vi "MaterialCharacterization.vi"(8 "error in":errorcluster) -> (0 "error out":errorcluster)   [LabVIEW 2013, in "MaterialCharacterization.lvlib"]
uses:
  MaterialCharacterization.lvlib
  Sources/Main/Options.ctl
  Sources/Main/Measurement-types.ctl
  Sources/Main/Main-actions.ctl
  Sources/Main/MC-Main.lvclass/MC-Main.ctl
  Sources/Main/Enqueue-modes.ctl
  Sources/UI/Pane-names.ctl
  Sources/Main/Write Measurement type.vi
  Sources/Main/Write Scan file path.vi
  Sources/Main/Read UI.vi
  Sources/UI/MC-UI.lvclass
  Sources/Main/MC-Main.lvclass
panel:
  in  "Measurement settings":bool
  in  "Select measurement":T1
  in  "Load configuration":bool
  in  "Stop":bool
  in  "Save configuration":bool
  in  "Activate":bool
  in  "Start":bool
  in  "Help":bool
  in  "View raw path":bool
  in  "SM1000 scan file":path
  in  "View scan file":bool
  in  "Options":T2
  out "Data table":string[][](table)
  out "Status":string caption="Status:"
  out "Action":string caption="Action:"
  # "Config"
  # "Exec"
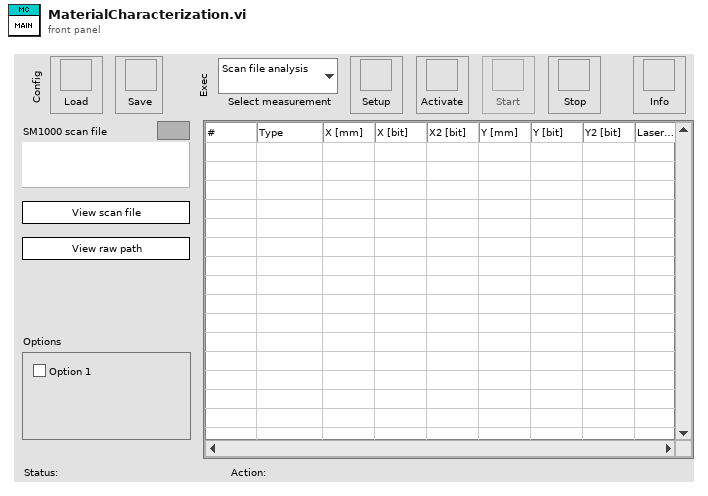
[diagram p1: front panel]
types:
  T1 = typedef "MaterialCharacterization.lvlib/MC-Main.lvclass/Measurement-types.ctl" = enum16{"Scan file analysis", "Thermal conductivity", "Laser reflection", "Combined"}
  T2 = typedef "MaterialCharacterization.lvlib/MC-Main.lvclass/Options.ctl" = cluster{"Option 1":bool}
  T3 = typedef "MaterialCharacterization.lvlib/MC-Main.lvclass/Main-actions.ctl" = enum16{"Idle", "Initialize", "Load configuration", "Save configuration", "Load file", "Edit settings", "View scan file", "View raw path", "Edit measurement settings", "Activate", "Start", "Stop", "Refresh display", "Exit"}
  T4 = typedef "MaterialCharacterization.lvlib/MC-Main.lvclass/Object-reference.ctl" = refnum<data-value>
  T5 = typedef "MaterialCharacterization.lvlib/MC-Main.lvclass/Enqueue-modes.ctl" = enum16{"Default", "Priority", "Flush"}
  T6 = typedef "MaterialCharacterization.lvlib/MC-UI.lvclass/Pane-names.ctl" = enum16{"Toolbar", "Help bar", "Toolbar lower border", "Center panel", "Main panel", "Settings panel", "Status bar upper border", "General state bar", "Information bar"}
  T7 = typedef "MaterialCharacterization.lvlib/MC-UI.lvclass/Panes-reference.ctl" = refnum<data-value>
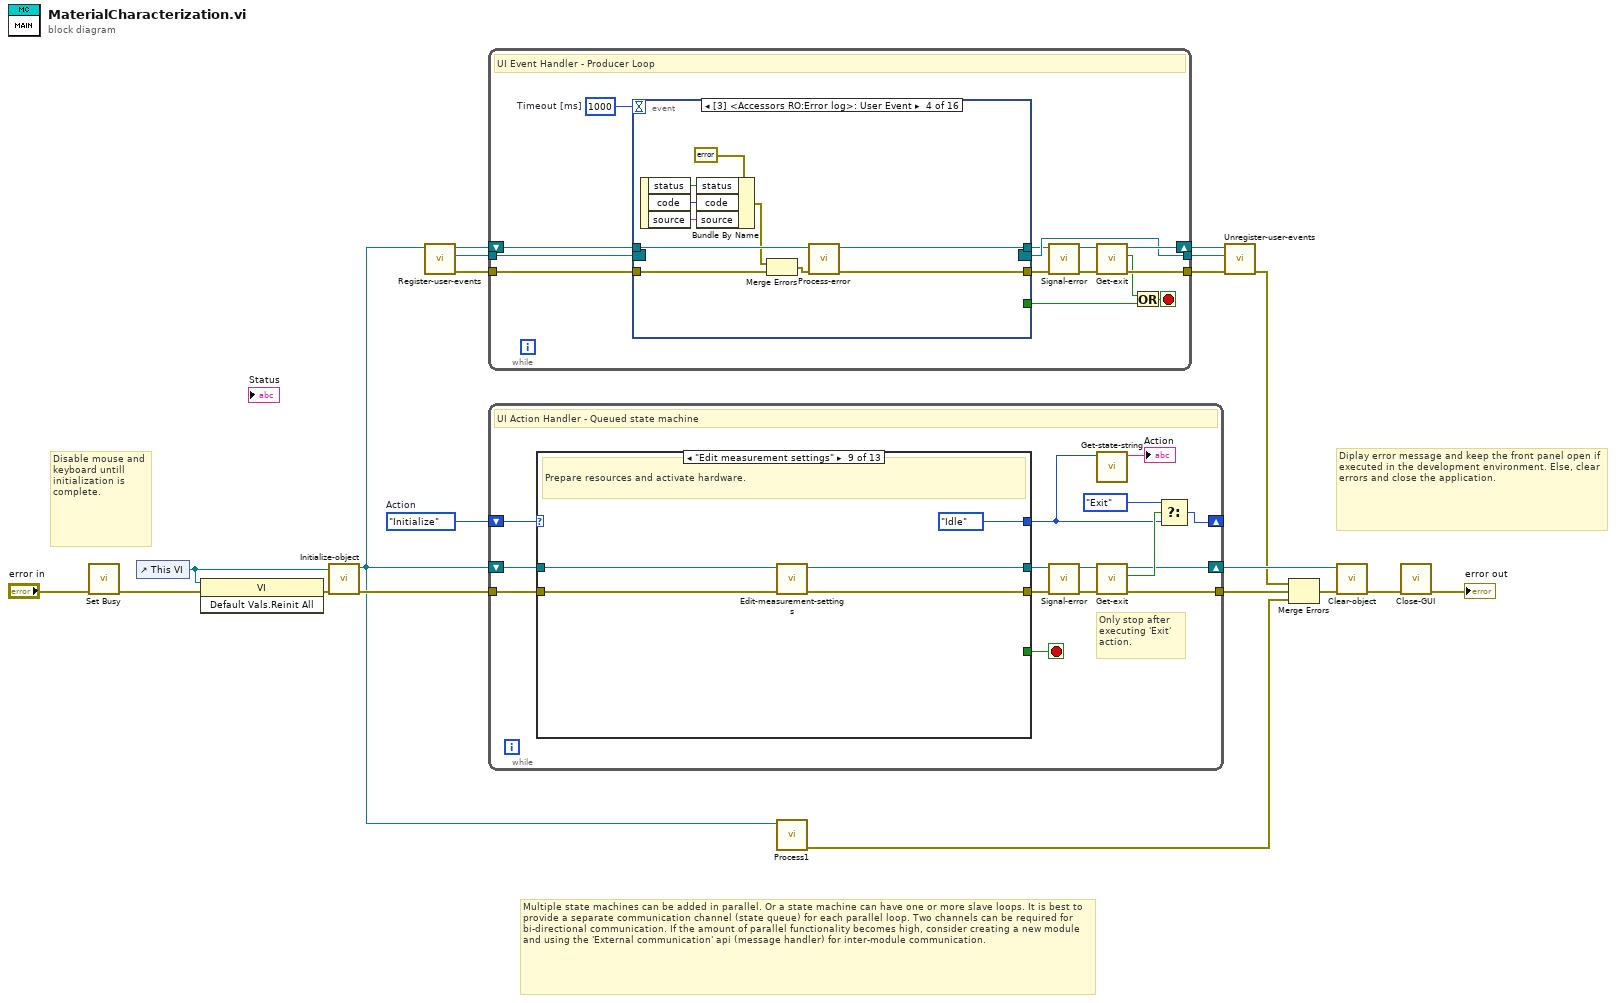
[diagram p0: block diagram]
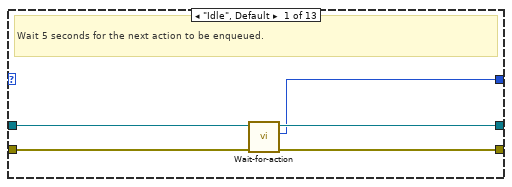
[diagram p2: hidden frame]
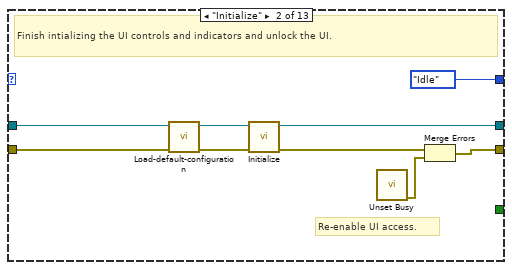
[diagram p3: hidden frame]
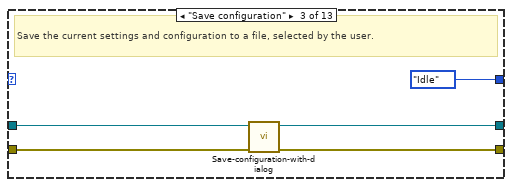
[diagram p4: hidden frame]
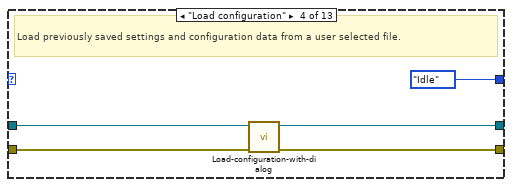
[diagram p5: hidden frame]
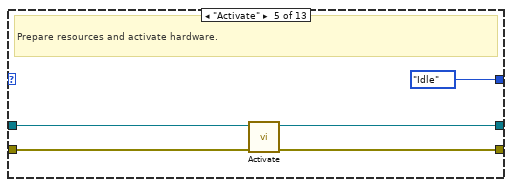
[diagram p6: hidden frame]
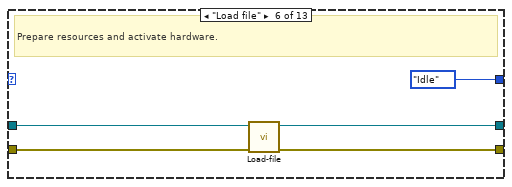
[diagram p7: hidden frame]
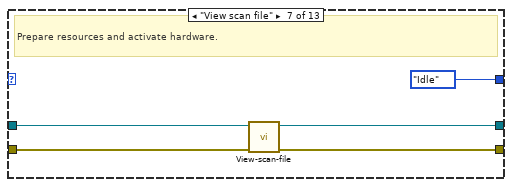
[diagram p8: hidden frame]
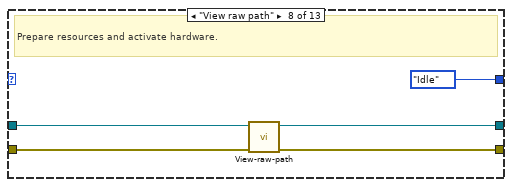
[diagram p9: hidden frame]
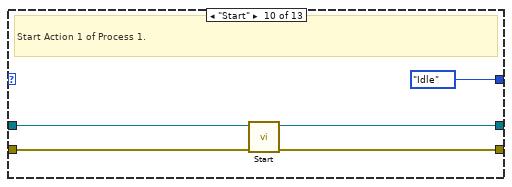
[diagram p10: hidden frame]
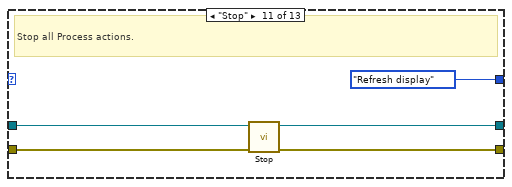
[diagram p11: hidden frame]
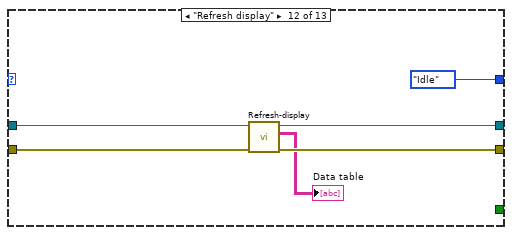
[diagram p12: hidden frame]
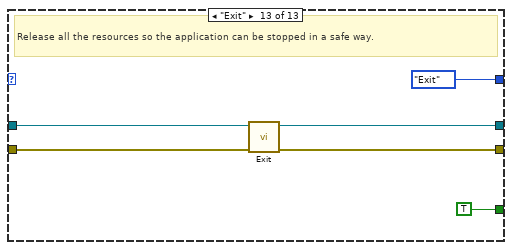
[diagram p13: hidden frame]
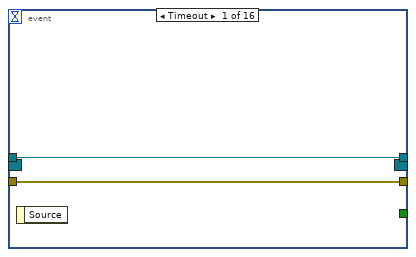
[diagram p14: hidden frame]
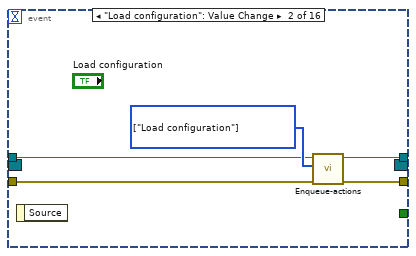
[diagram p15: hidden frame]
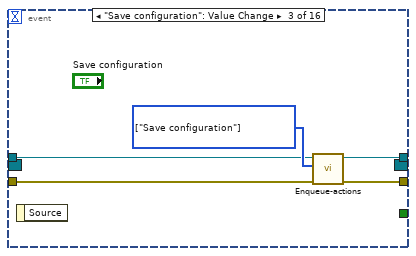
[diagram p16: hidden frame]
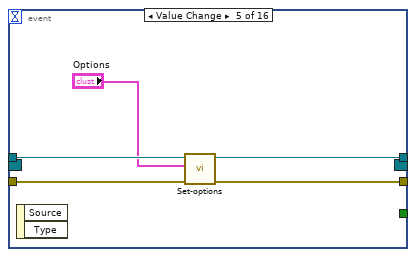
[diagram p17: hidden frame]
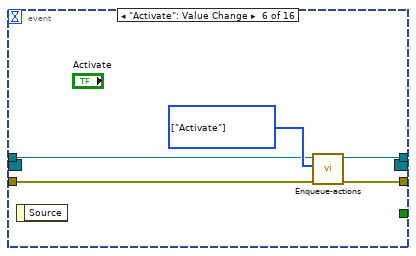
[diagram p18: hidden frame]
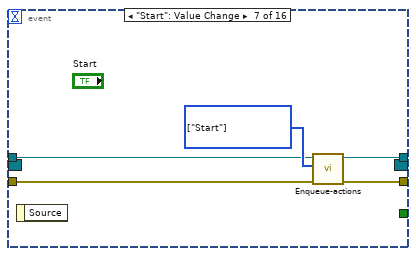
[diagram p19: hidden frame]
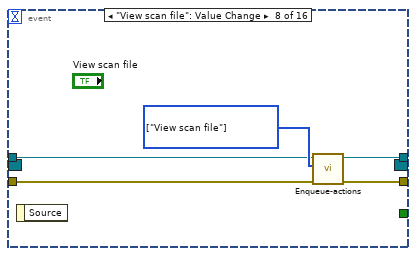
[diagram p20: hidden frame]
diagram:
  w20 = Main-actions."Initialize"  # Action
  # "Multiple state machines can be added in parallel. Or a state machine can have one or more slave loops. It is best to provide a separate communication channel (state queue) for each parallel loop. Two channels can be required for bi-directional communication. If the amount of parallel functionality becomes high, consider creating a new module and using the 'External communication' api (message handler) for inter-module communication."
  # "Disable mouse and keyboard untill initialization is complete."
  # "Diplay error message and keep the front panel open if executed in the development environment. Else, clear errors and close the application."
  n1 = call <vilib>:"Set Busy.vi"("error in (no error)"="error in") -> ("error out"=w3:errorcluster)  [unwired: 9 in, 1 out]
  n2 = control-ref of="This VI"() -> (w2:refnum<vi>)
  n3 = invoke class="VI" method="Default Vals.Reinit All"(reference=w2, error in=w3) -> (error out=w1:errorcluster)  [unwired: 1 in, 2 out]
  n4 = call "Initialize-object.vi"("Main VI ref"=w2, "error in (no error)"=w1) -> ("error out"=w13:errorcluster, "Object ref out"=w4:T4)  [unwired: 8 in]
  n5 = call "Register-user-events.vi"("Object ref in"=w4) -> ("error out"=w10:errorcluster, "Event registration"=w9:refnum<event-registration>, "Object ref out"=w11:T4)  [unwired: 8 in]
  n6 = while {
    shift-right: [w29] -> w6
    shift-left: w11 -> [w32]
    tunnel: w9 -> [w27]
    tunnel: [w26] -> w5
    tunnel: w10 -> [w33]
    tunnel: [w28] -> w8
    stop <- w23 stop-if-true
    w34 = 1000  # Timeout [ms]
    # "UI Event Handler - Producer Loop"
    n7 = event shown="[3] <Accessors RO:Error log>: User Event" {
      selector: w27 -> [_ _ _ _ _ _ _ _ _ _ _ _ _ _ _ _]
      dyn-events: [_ _ _ _ _ _ _ _ _ _ _ _ _ _ _ _] -> w26
      timeout: w34 -> [_ _ _ _ _ _ _ _ _ _ _ _ _ _ _ _]
      tunnel: w33 -> [w36 w41 w46 w54 w59 w66 w71 w76 w81 w86 w89 w92 w105 w108 w112 w156]
      tunnel: [w36 w40 w45 w53 w60 w65 w70 w75 w80 w85 w88 w95 w104 w108 w110 w161] -> w24
      tunnel: w32 -> [w35 w38 w43 w56 w58 w63 w68 w73 w78 w83 w91 w93 w102 w106 w113 w157]
      tunnel: [w35 w37 w42 w55 w61 w62 w67 w72 w77 w82 w90 w97 w101 w106 w111 w158] -> w25
      tunnel: [_ _ _ _ _ _ _ _ _ _ _ _ _ _ _ TRUE] -> w21
      event Timeout {
        n8 = event-data() -> ()  [unwired: 1 in, 1 out]
      }
      event "Load configuration": Value Change {
        w39 = T3[] [enum."Load configuration"] items=["Idle", "Initialize", "Load configuration", "Save configuration", "Load file", "Edit settings", "View scan file", "View raw path", "Edit measurement settings", "Activate", "Start", "Stop", "Refresh display", "Exit"] ("State array")
        n9 = event-data() -> ()  [unwired: 1 in, 1 out]
        n10 = call "Enqueue-actions.vi"("error in (no error)"=w41, "State array"=w39, "State queue in"=w38) -> ("error out"=w40:errorcluster, "State queue out"=w37:T4)  [unwired: 6 in, 1 out]
      }
      event "Save configuration": Value Change {
        w44 = T3[] [enum."Save configuration"] items=["Idle", "Initialize", "Load configuration", "Save configuration", "Load file", "Edit settings", "View scan file", "View raw path", "Edit measurement settings", "Activate", "Start", "Stop", "Refresh display", "Exit"] ("State array")
        n11 = event-data() -> ()  [unwired: 1 in, 1 out]
        n12 = call "Enqueue-actions.vi"("error in (no error)"=w46, "State array"=w44, "State queue in"=w43) -> ("error out"=w45:errorcluster, "State queue out"=w42:T4)  [unwired: 6 in, 1 out]
      }
      event User Event {
        n13 = event-data() -> ("status"=w51:bool, "code"=w50:i32, "source"=w49:string)  [unwired: 1 in]
        n14 = Bundle By Name(cluster=errorcluster {"status"=FALSE, "code"=0, "source"=""} ("error constant"), "status"=w51, "code"=w50, "source"=w49) -> (w47:errorcluster)
        n15 = Merge Errors(w47, w54) -> (w48:errorcluster)
        n16 = call "Process-error.vi"("error in (no error)"=w48, "Data in"=w56) -> ("error out"=w53:errorcluster, "Data out"=w55:T4)  [unwired: 8 in]
      }
      event Value Change {
        n17 = event-data() -> ()  [unwired: 1 in, 2 out]
        n18 = call "Set-options.vi"("error in (no error)"=w59, "Options"="Options", "Object ref in"=w58) -> ("error out"=w60:errorcluster, "Object ref out"=w61:T4)  [unwired: 7 in]
      }
      event "Activate": Value Change {
        w64 = T3[] [enum."Activate"] items=["Idle", "Initialize", "Load configuration", "Save configuration", "Load file", "Edit settings", "View scan file", "View raw path", "Edit measurement settings", "Activate", "Start", "Stop", "Refresh display", "Exit"] ("State array")
        n19 = event-data() -> ()  [unwired: 1 in, 1 out]
        n20 = call "Enqueue-actions.vi"("error in (no error)"=w66, "State array"=w64, "State queue in"=w63) -> ("error out"=w65:errorcluster, "State queue out"=w62:T4)  [unwired: 6 in, 1 out]
      }
      event "Start": Value Change {
        w69 = T3[] [enum."Start"] items=["Idle", "Initialize", "Load configuration", "Save configuration", "Load file", "Edit settings", "View scan file", "View raw path", "Edit measurement settings", "Activate", "Start", "Stop", "Refresh display", "Exit"] ("State array")
        n21 = event-data() -> ()  [unwired: 1 in, 1 out]
        n22 = call "Enqueue-actions.vi"("error in (no error)"=w71, "State array"=w69, "State queue in"=w68) -> ("error out"=w70:errorcluster, "State queue out"=w67:T4)  [unwired: 6 in, 1 out]
      }
      event "View scan file": Value Change {
        w74 = T3[] [enum."View scan file"] items=["Idle", "Initialize", "Load configuration", "Save configuration", "Load file", "Edit settings", "View scan file", "View raw path", "Edit measurement settings", "Activate", "Start", "Stop", "Refresh display", "Exit"] ("State array")
        n23 = event-data() -> ()  [unwired: 1 in, 1 out]
        n24 = call "Enqueue-actions.vi"("error in (no error)"=w76, "State array"=w74, "State queue in"=w73) -> ("error out"=w75:errorcluster, "State queue out"=w72:T4)  [unwired: 6 in, 1 out]
      }
      event "View raw path": Value Change {
        w79 = T3[] [enum."View raw path"] items=["Idle", "Initialize", "Load configuration", "Save configuration", "Load file", "Edit settings", "View scan file", "View raw path", "Edit measurement settings", "Activate", "Start", "Stop", "Refresh display", "Exit"] ("State array")
        n25 = event-data() -> ()  [unwired: 1 in, 1 out]
        n26 = call "Enqueue-actions.vi"("error in (no error)"=w81, "State array"=w79, "State queue in"=w78) -> ("error out"=w80:errorcluster, "State queue out"=w77:T4)  [unwired: 6 in, 1 out]
      }
      event "Measurement settings": Value Change {
        w84 = T3[] [enum."Edit measurement settings"] items=["Idle", "Initialize", "Load configuration", "Save configuration", "Load file", "Edit settings", "View scan file", "View raw path", "Edit measurement settings", "Activate", "Start", "Stop", "Refresh display", "Exit"] ("State array")
        n27 = event-data() -> ()  [unwired: 1 in, 1 out]
        n28 = call "Enqueue-actions.vi"("error in (no error)"=w86, "State array"=w84, "State queue in"=w83) -> ("error out"=w85:errorcluster, "State queue out"=w82:T4)  [unwired: 6 in, 1 out]
      }
      event Value Change {
        n29 = event-data() -> ()  [unwired: 1 in, 2 out]
        n30 = property class="MC-Main.lvclass"(reference=w91, error in=w89, "Accessors/Modifiers:V Measurement type"="Select measurement") -> (reference out=w90:T4, error out=w88:errorcluster)
      }
      event "SM1000 scan file": Value Change {
        w94 = T3[] [enum."Load file"] items=["Idle", "Initialize", "Load configuration", "Save configuration", "Load file", "Edit settings", "View scan file", "View raw path", "Edit measurement settings", "Activate", "Start", "Stop", "Refresh display", "Exit"] ("State array")
        n31 = event-data() -> ()  [unwired: 1 in, 2 out]
        n32 = property class="MC-Main.lvclass"(reference=w93, error in=w92, "Accessors/Modifiers:V Scan file path"="SM1000 scan file") -> (reference out=w98:T4, error out=w96:errorcluster)
        n33 = call "Enqueue-actions.vi"("error in (no error)"=w96, "State array"=w94, "State queue in"=w98) -> ("error out"=w95:errorcluster, "State queue out"=w97:T4)  [unwired: 6 in, 1 out]
      }
      event "Stop": Value Change {
        w103 = T3[] [enum."Stop"] items=["Idle", "Initialize", "Load configuration", "Save configuration", "Load file", "Edit settings", "View scan file", "View raw path", "Edit measurement settings", "Activate", "Start", "Stop", "Refresh display", "Exit"] ("State array")
        n34 = event-data() -> ()  [unwired: 1 in, 1 out]
        n35 = call "Enqueue-actions.vi"("Enqueue mode"=Enqueue-modes."Flush", "error in (no error)"=w105, "State array"=w103, "State queue in"=w102) -> ("error out"=w104:errorcluster, "State queue out"=w101:T4)  [unwired: 5 in, 1 out]
      }
      event "Help": Value Change {
        # "Toggle the visibility of the context help window."
        n36 = event-data() -> ()  [unwired: 1 in, 1 out]
        n37 = Control Help Window(1:"Help") -> ()  [unwired: 1 in]
      }
      event Menu Selection (User) {
        n38 = event-data() -> ("ItemTag"=w109:string)  [unwired: 1 in, 1 out]
        n39 = case shown="\"TOOLBAR\"" w109 {
          tunnel: w113 -> [w115 w119 w124 w129 w134 w139 w147 w154]
          tunnel: w112 -> [w114 w117 w122 w127 w132 w137 w143 w150]
          tunnel: [w115 w118 w123 w128 w133 w138 w146 w153] -> w111
          tunnel: [w114 w116 w121 w126 w131 w136 w145 w152] -> w110
          frame Default {
          }
          frame "LOAD_CONFIG" {
            w120 = T3[] [enum."Load configuration"] items=["Idle", "Initialize", "Load configuration", "Save configuration", "Load file", "Edit settings", "View scan file", "View raw path", "Edit measurement settings", "Activate", "Start", "Stop", "Refresh display", "Exit"] ("State array")
            n40 = call "Enqueue-actions.vi"("error in (no error)"=w117, "State array"=w120, "State queue in"=w119) -> ("error out"=w116:errorcluster, "State queue out"=w118:T4)  [unwired: 6 in, 1 out]
          }
          frame "SAVE_CONFIG" {
            w125 = T3[] [enum."Save configuration"] items=["Idle", "Initialize", "Load configuration", "Save configuration", "Load file", "Edit settings", "View scan file", "View raw path", "Edit measurement settings", "Activate", "Start", "Stop", "Refresh display", "Exit"] ("State array")
            n41 = call "Enqueue-actions.vi"("error in (no error)"=w122, "State array"=w125, "State queue in"=w124) -> ("error out"=w121:errorcluster, "State queue out"=w123:T4)  [unwired: 6 in, 1 out]
          }
          frame "ACTIVATE" {
            w130 = T3[] [enum."Activate"] items=["Idle", "Initialize", "Load configuration", "Save configuration", "Load file", "Edit settings", "View scan file", "View raw path", "Edit measurement settings", "Activate", "Start", "Stop", "Refresh display", "Exit"] ("State array")
            n42 = call "Enqueue-actions.vi"("error in (no error)"=w127, "State array"=w130, "State queue in"=w129) -> ("error out"=w126:errorcluster, "State queue out"=w128:T4)  [unwired: 6 in, 1 out]
          }
          frame "START" {
            w135 = T3[] [enum."Start"] items=["Idle", "Initialize", "Load configuration", "Save configuration", "Load file", "Edit settings", "View scan file", "View raw path", "Edit measurement settings", "Activate", "Start", "Stop", "Refresh display", "Exit"] ("State array")
            n43 = call "Enqueue-actions.vi"("error in (no error)"=w132, "State array"=w135, "State queue in"=w134) -> ("error out"=w131:errorcluster, "State queue out"=w133:T4)  [unwired: 6 in, 1 out]
          }
          frame "STOP" {
            w140 = T3[] [enum."Stop"] items=["Idle", "Initialize", "Load configuration", "Save configuration", "Load file", "Edit settings", "View scan file", "View raw path", "Edit measurement settings", "Activate", "Start", "Stop", "Refresh display", "Exit"] ("State array")
            n44 = call "Enqueue-actions.vi"("error in (no error)"=w137, "State array"=w140, "State queue in"=w139) -> ("error out"=w136:errorcluster, "State queue out"=w138:T4)  [unwired: 6 in, 1 out]
          }
          frame "TOOLBAR" {
            n45 = property class="MC-Main.lvclass"(reference=w147, error in=w143) -> (reference out=w146:T4, error out=w144:errorcluster, "Accessors RO:UI"=w142:T7)
            n46 = call "Toggle-pane.vi"("error in (no error)"=w144, "Pane"=Pane-names."Toolbar", "Panes in"=w142) -> ("error out"=w145:errorcluster)  [unwired: 6 in, 2 out]
          }
          frame "SETTINGS" {
            n47 = property class="MC-Main.lvclass"(reference=w154, error in=w150) -> (reference out=w153:T4, error out=w151:errorcluster, "Accessors RO:UI"=w149:T7)
            n48 = call "Toggle-pane.vi"("error in (no error)"=w151, "Pane"=Pane-names."Settings panel", "Panes in"=w149) -> ("error out"=w152:errorcluster)  [unwired: 6 in, 2 out]
          }
        }
      }
      event Panel Close? {
        w159 = T3[] [enum."Stop", enum."Exit"] items=["Idle", "Initialize", "Load configuration", "Save configuration", "Load file", "Edit settings", "View scan file", "View raw path", "Edit measurement settings", "Activate", "Start", "Stop", "Refresh display", "Exit"] ("State array")
        # "Discard event, to allow time to exit in a safe way."
        # "The user can stop the program by pressing the X in the window corner."
        n49 = event-data() -> ()  [unwired: 1 in, 1 out]
        n50 = call "Enqueue-actions.vi"("Enqueue mode"=Enqueue-modes."Flush", "error in (no error)"=w156, "State array"=w159, "State queue in"=w157) -> ("error out"=w161:errorcluster, "State queue out"=w158:T4)  [unwired: 5 in, 1 out]
        n51 = event-data("Discard?"=TRUE ("Exit?")) -> ()  [unwired: 1 in, 1 out]
      }
    }
    n52 = call "Signal-error.vi"("error in (no error)"=w24, "Data in"=w25) -> ("error out"=w31:errorcluster, "Data out"=w30:T4)  [unwired: 8 in]
    n53 = call "Get-exit.vi"("error in (no error)"=w31, "Object ref in"=w30) -> ("error out"=w28:errorcluster, "Exit?"=w22:bool, "Object ref out"=w29:T4)  [unwired: 7 in]
    n54 = Or(x=w22, y=w21) -> (x .or. y?=w23:bool)
  }
  n55 = while {
    shift-right: [w171] -> _
    shift-left: w20 -> [w174]
    shift-right: [w165] -> w14
    shift-left: w4 -> [w176]
    tunnel: w13 -> [w175]
    tunnel: [w164] -> w19
    stop <- w177 stop-if-true
    # "Only stop after executing 'Exit' action."
    # "UI Action Handler - Queued state machine"
    n56 = case shown="\"Edit measurement settings\"" w174 {
      tunnel: [w179 Main-actions."Idle" ("States") Main-actions."Idle" ("States") Main-actions."Idle" ("States") Main-actions."Idle" ("States") Main-actions."Idle" ("States") Main-actions."Idle" ("States") Main-actions."Idle" ("States") Main-actions."Idle" ("States") Main-actions."Idle" ("States") Main-actions."Refresh display" ("States") Main-actions."Idle" ("States") Main-actions."Exit" ("States")] -> w168
      tunnel: [_ _ _ _ _ _ _ _ _ _ _ _ TRUE] -> w177
      tunnel: w176 -> [w181 w188 w195 w200 w205 w210 w215 w220 w225 w231 w235 w241 w246]
      tunnel: [w180 w189 w194 w199 w204 w209 w214 w219 w224 w229 w233 w239 w243] -> w166
      tunnel: w175 -> [w178 w187 w193 w198 w202 w207 w212 w217 w222 w230 w234 w240 w245]
      tunnel: [w182 w184 w192 w197 w203 w208 w213 w218 w223 w228 w232 w238 w244] -> w167
      frame "Idle", Default {
        # "Wait 5 seconds for the next action to be enqueued."
        n57 = call "Wait-for-action.vi"("error in (no error)"=w178, "Object ref in"=w181) -> ("error out"=w182:errorcluster, "Next action"=w179:T3, "Object ref out"=w180:T4)  [unwired: 7 in]
      }
      frame "Initialize" {
        # "Re-enable UI access."
        # "Finish intializing the UI controls and indicators and unlock the UI."
        n58 = call "Load-default-configuration.vi"("error in (no error)"=w187, "Object ref in"=w188) -> ("error out"=w186:errorcluster, "Object ref out"=w185:T4)  [unwired: 8 in]
        n59 = call "Initialize.vi"("error in (no error)"=w186, "Object ref in"=w185) -> ("error out"=w183:errorcluster, "Object ref out"=w189:T4)  [unwired: 8 in]
        n60 = call <vilib>:"Unset Busy.vi"() -> ("error out"=w190:errorcluster)  [unwired: 11 in]
        n61 = Merge Errors(w183, w190) -> (w184:errorcluster)
      }
      frame "Save configuration" {
        # "Save the current settings and configuration to a file, selected by the user."
        n62 = call "Save-configuration-with-dialog.vi"("error in (no error)"=w193, "Object ref in"=w195) -> ("error out"=w192:errorcluster, "Object ref out"=w194:T4)  [unwired: 7 in, 1 out]
      }
      frame "Load configuration" {
        # "Load previously saved settings and configuration data from a user selected file."
        n63 = call "Load-configuration-with-dialog.vi"("error in (no error)"=w198, "Object ref in"=w200) -> ("error out"=w197:errorcluster, "Object ref out"=w199:T4)  [unwired: 8 in]
      }
      frame "Activate" {
        # "Prepare resources and activate hardware."
        n64 = call "Activate.vi"("error in (no error)"=w202, "Object ref in"=w205) -> ("error out"=w203:errorcluster, "Object ref out"=w204:T4)  [unwired: 8 in]
      }
      frame "Load file" {
        # "Prepare resources and activate hardware."
        n65 = call "Load-file.vi"("error in (no error)"=w207, "Object ref in"=w210) -> ("error out"=w208:errorcluster, "Object ref out"=w209:T4)  [unwired: 8 in]
      }
      frame "View scan file" {
        # "Prepare resources and activate hardware."
        n66 = call "View-scan-file.vi"("error in (no error)"=w212, "Object ref in"=w215) -> ("error out"=w213:errorcluster, "Object ref out"=w214:T4)  [unwired: 8 in]
      }
      frame "View raw path" {
        # "Prepare resources and activate hardware."
        n67 = call "View-raw-path.vi"("error in (no error)"=w217, "Object ref in"=w220) -> ("error out"=w218:errorcluster, "Object ref out"=w219:T4)  [unwired: 8 in]
      }
      frame "Edit measurement settings" {
        # "Prepare resources and activate hardware."
        n68 = call "Edit-measurement-settings.vi"("error in (no error)"=w222, "Object ref in"=w225) -> ("error out"=w223:errorcluster, "Object ref out"=w224:T4)  [unwired: 8 in]
      }
      frame "Start" {
        # "Start Action 1 of Process 1."
        n69 = call "Start.vi"("error in (no error)"=w230, "Object ref in"=w231) -> ("error out"=w228:errorcluster, "Object ref out"=w229:T4)  [unwired: 8 in]
      }
      frame "Stop" {
        # "Stop all Process actions."
        n70 = call "Stop.vi"("error in (no error)"=w234, "Object ref in"=w235) -> ("error out"=w232:errorcluster, "Object ref out"=w233:T4)  [unwired: 8 in]
      }
      frame "Refresh display" {
        n71 = call "Refresh-display.vi"("error in (no error)"=w240, "Object ref in"=w241) -> ("error out"=w238:errorcluster, "Array"=→"Data table":string[][], "Object ref out"=w239:T4)  [unwired: 7 in]
      }
      frame "Exit" {
        # "Release all the resources so the application can be stopped in a safe way."
        n72 = call "Exit.vi"("error in (no error)"=w245, "Object ref in"=w246) -> ("error out"=w244:errorcluster, "Object ref out"=w243:T4)  [unwired: 8 in]
      }
    }
    n73 = call "Signal-error.vi"("error in (no error)"=w167, "Data in"=w166) -> ("error out"=w173:errorcluster, "Data out"=w172:T4)  [unwired: 8 in]
    n74 = call "Get-state-string.vi"("States"=w168) -> ("State string"=→"Action":string)  [unwired: 10 in]
    n75 = call "Get-exit.vi"("error in (no error)"=w173, "Object ref in"=w172) -> ("error out"=w164:errorcluster, "Exit?"=w169:bool, "Object ref out"=w165:T4)  [unwired: 7 in]
    n76 = Select(t=Main-actions."Exit" ("States"), s=w169, f=w168) -> (s? t:f=w171:T3)
  }
  n77 = call "Process1.vi"("Object ref in"=w4) -> ("error out"=w12:errorcluster)  [unwired: 9 in, 1 out]
  n78 = call "Unregister-user-events.vi"("error in (no error)"=w8, "Event registration"=w5, "Object ref in"=w6) -> ("error out"=w7:errorcluster)  [unwired: 7 in, 1 out]
  n79 = Merge Errors(w7, w19, w12) -> (w17:errorcluster)
  n80 = call "Clear-object.vi"("error in (no error)"=w17, "Object ref in"=w14) -> ("error out"=w16:errorcluster)  [unwired: 9 in]
  n81 = call "Close-GUI.vi"("error in (no error)"=w16) -> ("error out"=→"error out":errorcluster)  [unwired: 10 in]
